vi "PCO_SetUserPowerDownTime.vi"(8 "error in (no error)":errorcluster {"code" format="%x"}, 10 "dwPowerDownTime":u32, 11 "ph":u64) -> (0 "error out":errorcluster {"code" format="%x"}, 2 "ErrorMessage":i32 format="%x", 3 "ph out":u64)   [LabVIEW 2019, in "SDK.lvlib" / "TimingControl.lvlib"]
doc: "<b>Description:</b>\nThis function does set the power down threshold time for power down mode [user]. If the exposure time is greater than the selected threshold time the sensor is switched into a special low energy mode to reduce dark current effects. Because the wake-up of the camera from this special mode does need some time the value of the wPowerDownTime should not be less then 1000 ms, which is also the default value when power down mode is [auto].\n\n<b>Supported camera type:</b>\npco.1600, pco.2000, pco.4000\n\n<b>Descriptor dependency:</b>\nwPowerDownModeDESC"
uses:
  TimingControl.lvlib
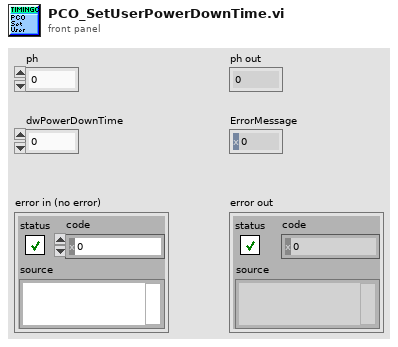
[diagram p1: front panel]
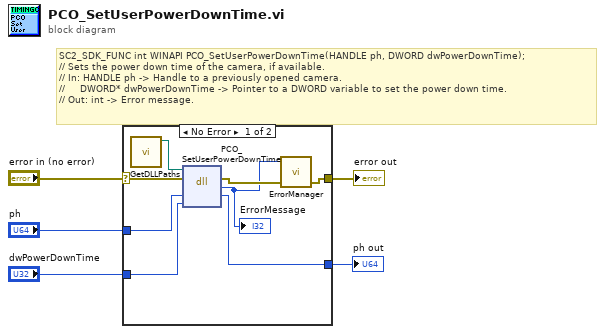
[diagram p0: block diagram]
diagram:
  # "SC2_SDK_FUNC int WINAPI PCO_SetUserPowerDownTime(HANDLE ph, DWORD dwPowerDownTime);\n// Sets the power down time of the camera, if available.\n// In: HANDLE ph -> Handle to a previously opened camera.\n//     DWORD* dwPowerDownTime -> Pointer to a DWORD variable to set the power down time.\n// Out: int -> Error message."
  n1 = case shown="No Error" "error in (no error)" {
    selector: "error in (no error)" -> [w10 w15]
    tunnel: "ph" -> [w13 w14]
    tunnel: [w12 w14] -> w4
    tunnel: "dwPowerDownTime" -> [w11 _]
    tunnel: [w8 w15] -> w2
    frame No Error {
      n2 = call "GetDLLPaths.vi"() -> ("SC2_Cam_Path"=w6:path)  [unwired: 9 in, 2 out]
      n3 = dll-call lib="?" fn="PCO_SetUserPowerDownTime"(path in=w6, error in=w10, "ph"=w13, "dwPowerDownTime"=w11) -> (error out=w9:errorcluster, "return type"=w7:i32, "ph"=w12:u64)  [unwired: 2 in, 1 out]
      "ErrorMessage" <- w7
      n4 = call "ErrorManager.vi"("error in (no error)"=w9, "error code"=w7) -> ("error out"=w8:errorcluster)  [unwired: 3 in]
    }
    frame Error {
    }
  }
  "ph out" <- w4
  "error out" <- w2
